vi "Update Waveform Increment.vi"(8 "error in (no error)":errorcluster, 10 "Increment":u32, 11 "Data in":T1) -> (0 "error out":errorcluster)   [LabVIEW 2017, in "Test Bench.lvlib"]
uses:
  Test Bench.lvlib
  Scan Engine Variables.ctl
  <instrlib>/_niInstr/FIFO Register Bus/v1/Host/niInstr FIFO Register Bus v1 Host.lvclass
  C:/Program Files (x86)/National Instruments/LabVIEW 2017/instr.lib/_niInstr/Instruction Framework/v1/Host/Instruction Target/niInstr Instruction Target v1 Host.lvclass
  <instrlib>/_niInstr/Instruction Framework/v1/Host/Instruction Framework Context/niInstr Instruction Framework Context v1 Host.lvclass
  <instrlib>/_niInstr/Instruction Framework/v1/Host/Instruction Target/niInstr Instruction Target v1 Host.lvclass
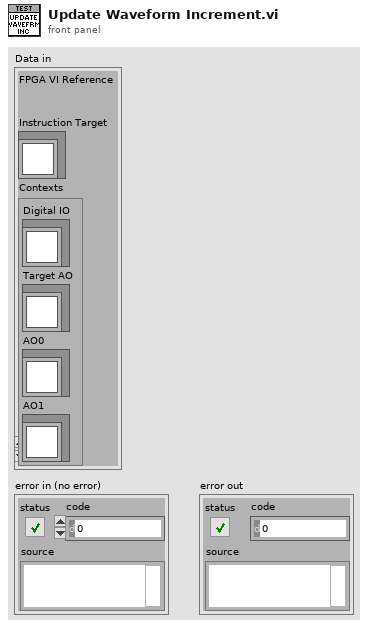
[diagram p1: front panel]
types:
  T1 = typedef "Test Bench.lvlib/Scan Engine Variables.ctl" = cluster{"FPGA VI Reference":refnum<k20>, "Instruction Target":refnum<class "niInstr FIFO Register Bus v1 Host.lvclass">, "Contexts":cluster{"Digital IO":refnum<class "niInstr Instruction Framework Context v1 Host.lvclass">, "Target AO":refnum<class "niInstr Instruction Framework Context v1 Host.lvclass">, "AO0":refnum<class "niInstr Instruction Framework Context v1 Host.lvclass">, "AO1":refnum<class "niInstr Instruction Framework Context v1 Host.lvclass">}}
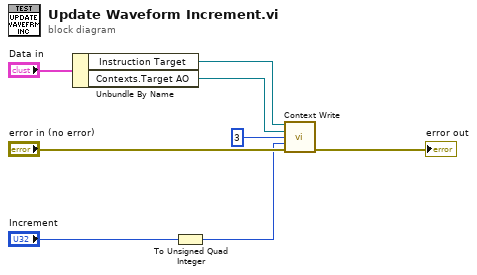
[diagram p0: block diagram]
diagram:
  n1 = Unbundle By Name("Data in") -> ("Instruction Target"=w6:refnum<class "niInstr FIFO Register Bus v1 Host.lvclass">, "Contexts.Target AO"=w5:refnum<class "niInstr Instruction Framework Context v1 Host.lvclass">)
  n2 = To Unsigned Quad Integer(1:"Increment") -> (0:w1:u64)
  n3 = call <instrlib>:"Context Write.vi"("instruction target in"=w6, "context in"=w5, "address"=u64 3, "data"=w1, "error in"="error in (no error)") -> ("error out"=→"error out":errorcluster)  [unwired: 8 in, 2 out]
